vi "Keithley3Fres.vi"(2 "Delay":dbl, 3 "Average Measurements":dbl, 4 "VISA resource name":refnum<visa-resource-name>) -> (1 "Resistance Array":dbl[](array[numeric]))   [LabVIEW 2014]
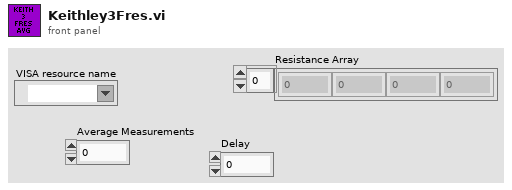
[diagram p1: front panel]
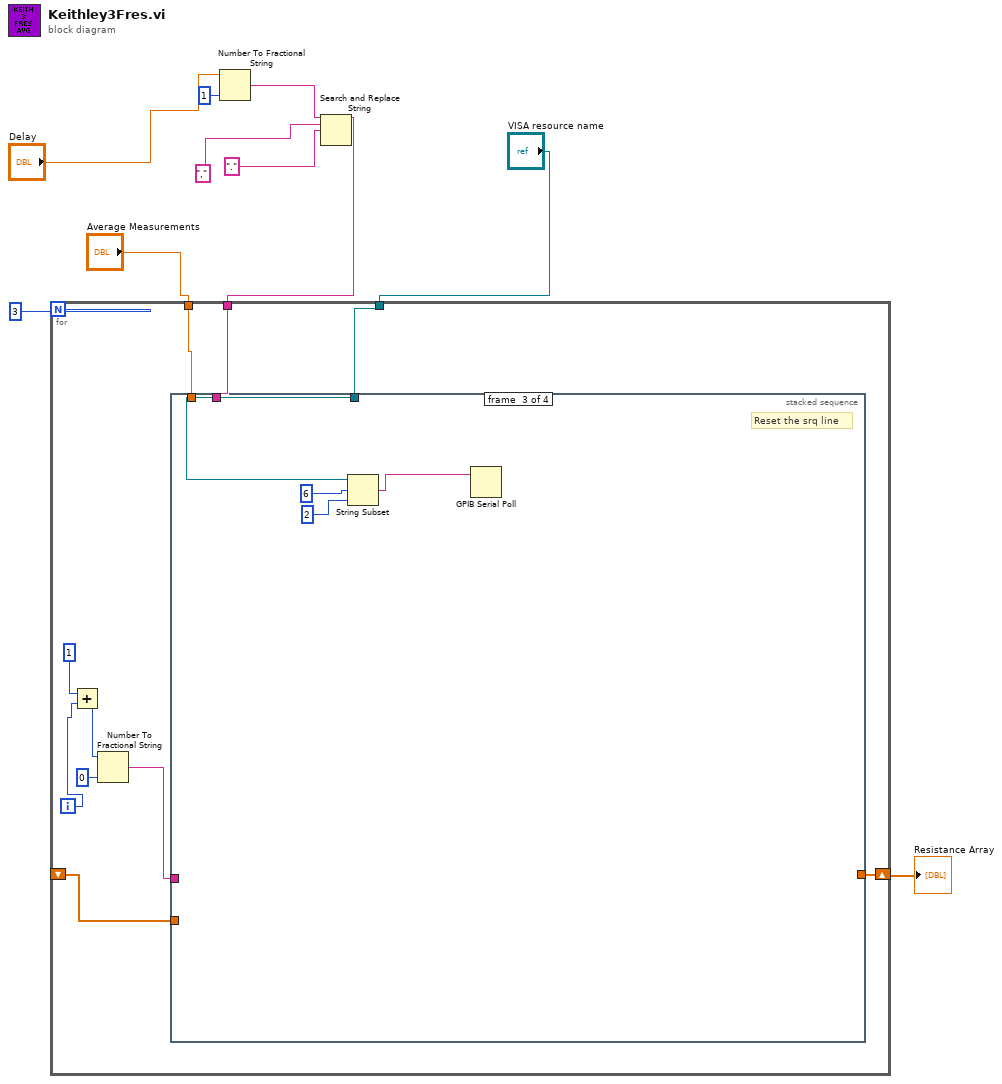
[diagram p0: block diagram]
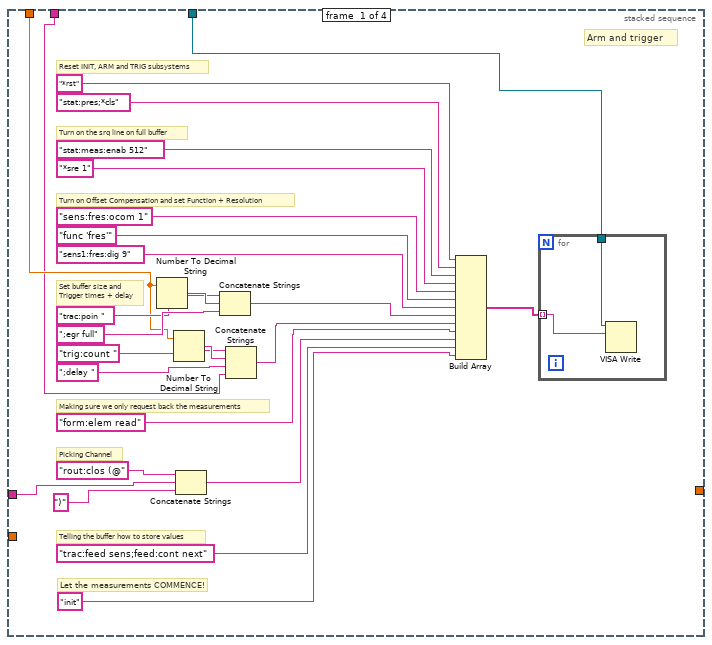
[diagram p2: hidden frame]
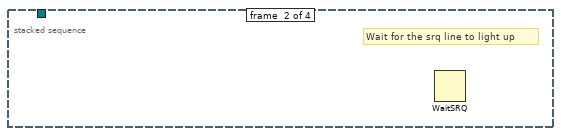
[diagram p3: hidden frame]
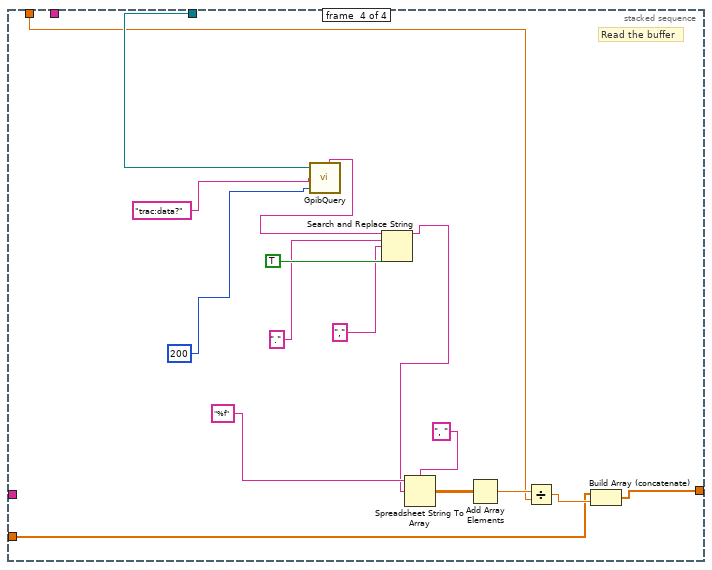
[diagram p4: hidden frame]
diagram:
  n1 = Number To Fractional String(number="Delay", precision (6)=i16 1) -> (F-format string=w10:string)  [unwired: 2 in]
  n2 = Search and Replace String(input string=w10, search string=",", replace string=".") -> (result string=w4:string)  [unwired: 5 in, 3 out]
  n3 = for {
    N: 3 -> [_]
    tunnel: "VISA resource name" -> [w20]
    tunnel: w4 -> [w19]
    tunnel: "Average Measurements" -> [w18]
    shift-right: [w13] -> w6
    shift-left: _ -> [w12]
    i -> [w16]
    n4 = Add(x=1, y=w16) -> (x+y=w15:i32)
    n5 = Number To Fractional String(number=w15, precision (6)=i16 0) -> (F-format string=w14:string)  [unwired: 2 in]
    n6 = stacked-sequence {
      tunnel: w20 -> [w46 _ w50 w60]
      tunnel: w18 -> [w33 _ _ w56]
      tunnel: w19 -> [w32 _ _ _]
      tunnel: w14 -> [w21 _ _ _]
      tunnel: [_ _ _ w54] -> w13
      tunnel: w12 -> [_ _ _ w53]
      frame #0 {
        # "Let the measurements COMMENCE!"
        # "Telling the buffer how to store values"
        # "Picking Channel"
        # "Making sure we only request back the measurements"
        # "Set buffer size and \nTrigger times + delay"
        # "Turn on Offset Compensation and set Function + Resolution"
        # "Turn on the srq line on full buffer"
        # "Reset INIT, ARM and TRIG subsystems"
        # "Arm and trigger"
        n7 = Number To Decimal String(number=w33) -> (decimal integer string=w39:string)  [unwired: 1 in]
        n8 = Number To Decimal String(number=w33) -> (decimal integer string=w42:string)  [unwired: 1 in]
        n9 = Concatenate Strings("rout:clos (@", w21, ")") -> (w25:string)
        n10 = Concatenate Strings("trac:poin ", w39, ";egr full") -> (w28:string)
        n11 = Concatenate Strings("trig:count ", w42, ";delay ", w32) -> (w27:string)
        n12 = Build Array("*rst", "stat:pres;*cls", "stat:meas:enab 512", "*sre 1", "sens:fres:ocom 1", "func 'fres'", "sens1:fres:dig 9", w28, w27, "form:elem read", w25, "trac:feed sens;feed:cont next", "init") -> (w22:string[])
        n13 = for {
          tunnel: w46 -> [w48]
          tunnel: w22 -> [w47] mode=indexing
          n14 = VISA Write(VISA resource name=w48, write buffer=w47) -> ()  [unwired: 1 in, 3 out]
        }
      }
      frame #1 {
        # "Wait for the srq line to light up"
        n15 = WaitSRQ() -> ()  [unwired: 2 in, 3 out]
      }
      frame #2 {
        # "Reset the srq line"
        n16 = String Subset(string=w50, offset (0)=6, length (rest)=2) -> (substring=w49:string)
        n17 = GPIB Serial Poll(0:w49) -> ()  [unwired: 1 in, 3 out]
      }
      frame #3 {
        # "Read the buffer"
        n18 = call "GpibQuery.vi"("Wait (ms)"=200, "Command"="trac:data?", "VISA resource name"=w60) -> ("Return Value"=w57:string)  [unwired: 1 in, 4 out]
        n19 = Search and Replace String(replace all?=TRUE ("replace all? (F)"), input string=w57, search string=".", replace string=",") -> (result string=w64:string)  [unwired: 4 in, 3 out]
        n20 = Spreadsheet String To Array(delimiter (Tab)=", ", format string="%f", spreadsheet string=w64) -> (array=w62:dbl[][])  [unwired: 1 in]
        n21 = Add Array Elements(numeric array=w62) -> (sum=w61:dbl)
        n22 = Divide(x=w61, y=w56) -> (x/y=w55:dbl)
        n23 = Build Array (concatenate)(w53, w55) -> (w54:dbl[])
      }
    }
  }
  "Resistance Array" <- w6
